vi "Framework.Initialize.vi"(8 "error in (no error)":errorcluster, 10 "Framework Configuration":refnum<class "Framework Configuration.lvclass">, 11 "Framework type":refnum<class "Framework.lvclass">) -> (0 "error out":errorcluster, 3 "Framework out":refnum<class "Framework.lvclass">)   [LabVIEW 2017, in "DSF Core.lvlib" / "Framework.lvclass"]
uses:
  Framework.lvclass
  Shared/Classes/Framework/Framework Configuration.lvclass
  Shared/Classes/Framework/Framework Configuration.lvclass/Framework Configuration.ctl
  Framework.lvclass/Framework.ctl
  Status/Framework Status.lvclass
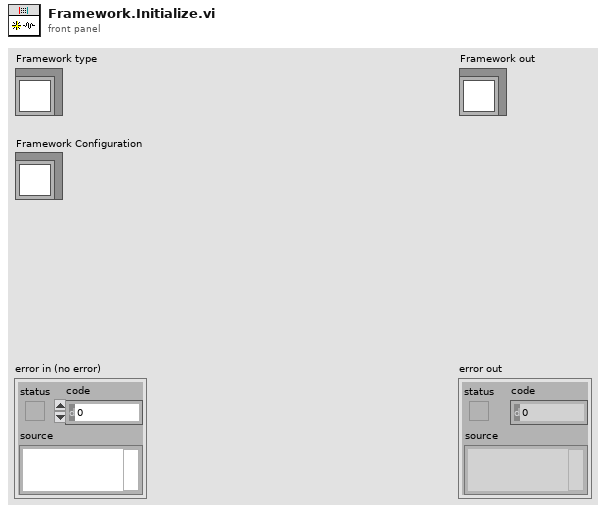
[diagram p1: front panel]
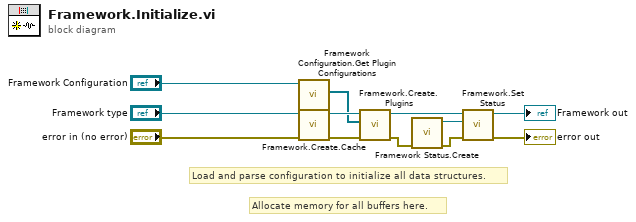
[diagram p0: block diagram]
diagram:
  # "Allocate memory for all buffers here."
  # "Load and parse configuration to initialize all data structures."
  n1 = call "Framework Configuration.Get Plugin Configurations.vi"("Framework Configuration in"="Framework Configuration") -> ("Plugin Configurations"=w7:refnum<class "Plugin Configuration.lvclass">[])  [unwired: 9 in, 1 out]
  n2 = call "Framework.Create.Cache.vi"("error in (no error)"="error in (no error)", "Framework in"="Framework type") -> ("error out"=w8:errorcluster, "Framework out"=w9:refnum<class "Framework.lvclass">)  [unwired: 8 in]
  n3 = call "Framework.Create.Plugins.vi"("error in (no error)"=w8, "Plugin Configurations"=w7, "Framework in"=w9) -> ("error out"=w6:errorcluster, "Framework out"=w3:refnum<class "Framework.lvclass">)  [unwired: 6 in, 1 out]
  n4 = call "Framework Status.Create.vi"("error in (no error)"=w6) -> ("error out"=→"error out":errorcluster, "Framework Status"=w4:refnum<class "Framework Status.lvclass">)  [unwired: 9 in]
  n5 = call "Framework.Set Status.vi"("Status"=w4, "Framework in"=w3) -> ("Framework out"=→"Framework out":refnum<class "Framework.lvclass">)  [unwired: 9 in]
